vi "员工管理测试程序.vi"() -> (1 "员工姓名":string, 2 "员工ID":string)   [LabVIEW 2013]
panel:
  out "权限":bool
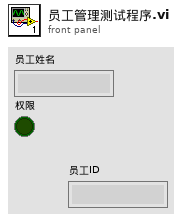
[diagram p1: front panel]
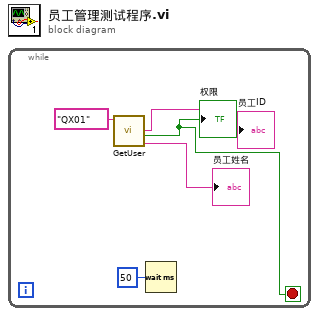
[diagram p0: block diagram]
diagram:
  n1 = while {
    stop <- w2 stop-if-true
    n2 = call "GetUser.vi"("权限"="QX01") -> ("员工姓名"=→"员工姓名":string, "权限"=w2:bool, "员工ID"=→"员工ID":string)  [unwired: 8 in]
    "权限" <- w2
    n3 = Wait (ms)(milliseconds to wait=u32 50 ("等待时间（毫秒）")) -> ()  [unwired: 1 out]
  }
